vi "TempSim SubVI.vi"(0 "Stopped Boolean":refnum<vi>, 1 "Temperature Queue in":refnum<queue>, 2 "Frequency":dbl, 5 "error in (no error)":errorcluster, 6 "LightCases in":T1, 7 "Temperatures in":T4, 8 "TemperatureData in":T2) -> (10 "TemperatureData out":T2, 11 "Stop loop?":bool, 12 "LightCases out":T1, 13 "Temperatures out":T4, 14 "F0 Temp Chart":dbl(graph), 15 "F0 Gain":dbl, 16 "Kinti hõmérséklet":dbl, 17 "F1 Temp Chart":dbl(graph), 18 "F1 Gain":dbl, 19 "error out":errorcluster)   [LabVIEW 2014]
uses:
  Types/TemperatureArray.ctl
  Types/TemperatureControlData.ctl
  Types/HeatingMode.ctl
  Types/LightCases.ctl
  Types/FVGFuncts.ctl
  <vilib>/express/express arith-compare/Formula/XNode/ExpressFormulaBlockNode.xnode
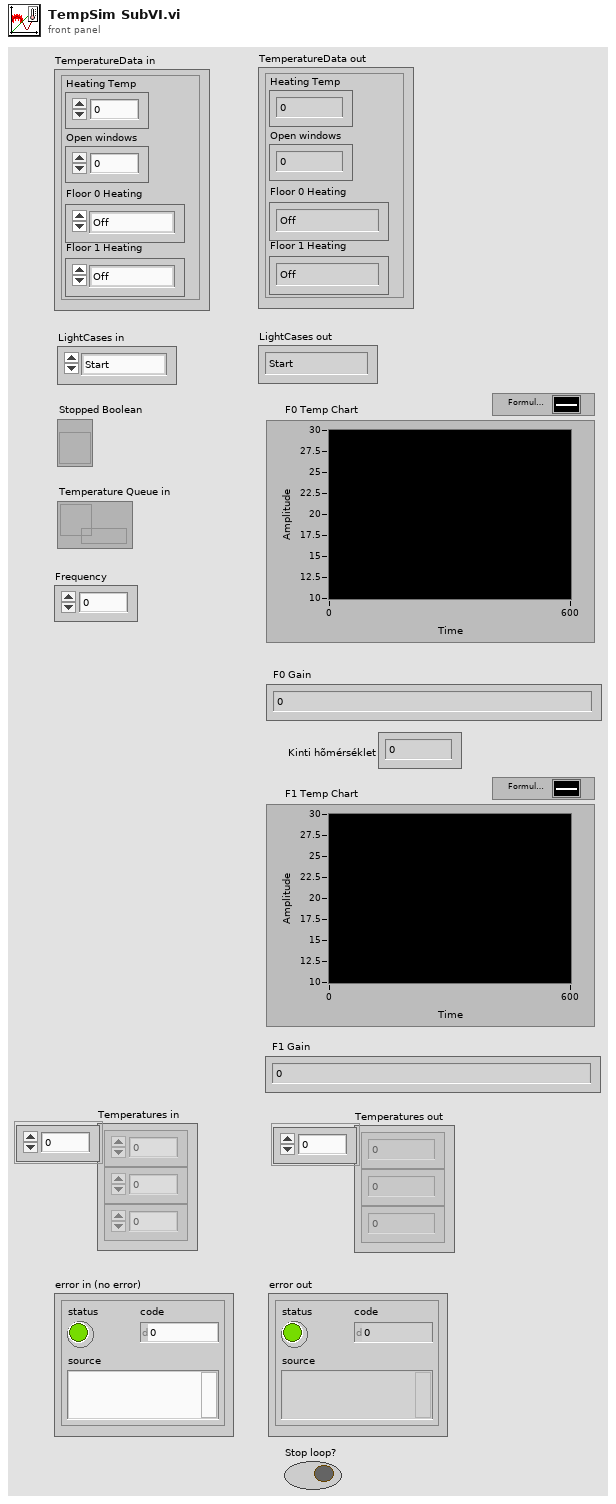
[diagram p1: front panel]
types:
  T1 = typedef "LightCases.ctl" = enum16{"Start", "Update", "Stop"}
  T2 = typedef "TemperatureControlData.ctl" = cluster{"Open windows":dbl, "Floor 0 Heating":T3, "Floor 1 Heating":T3, "Heating Temp":dbl}
  T3 = typedef "HeatingMode.ctl" = enum16{"Off", "Heating", "Cooling"}
  T4 = typedef "TemperatureArray.ctl" = dbl[]
  T5 = typedef "FVGFuncts.ctl" = enum16{"Init", "Set Data", "Get Data"}
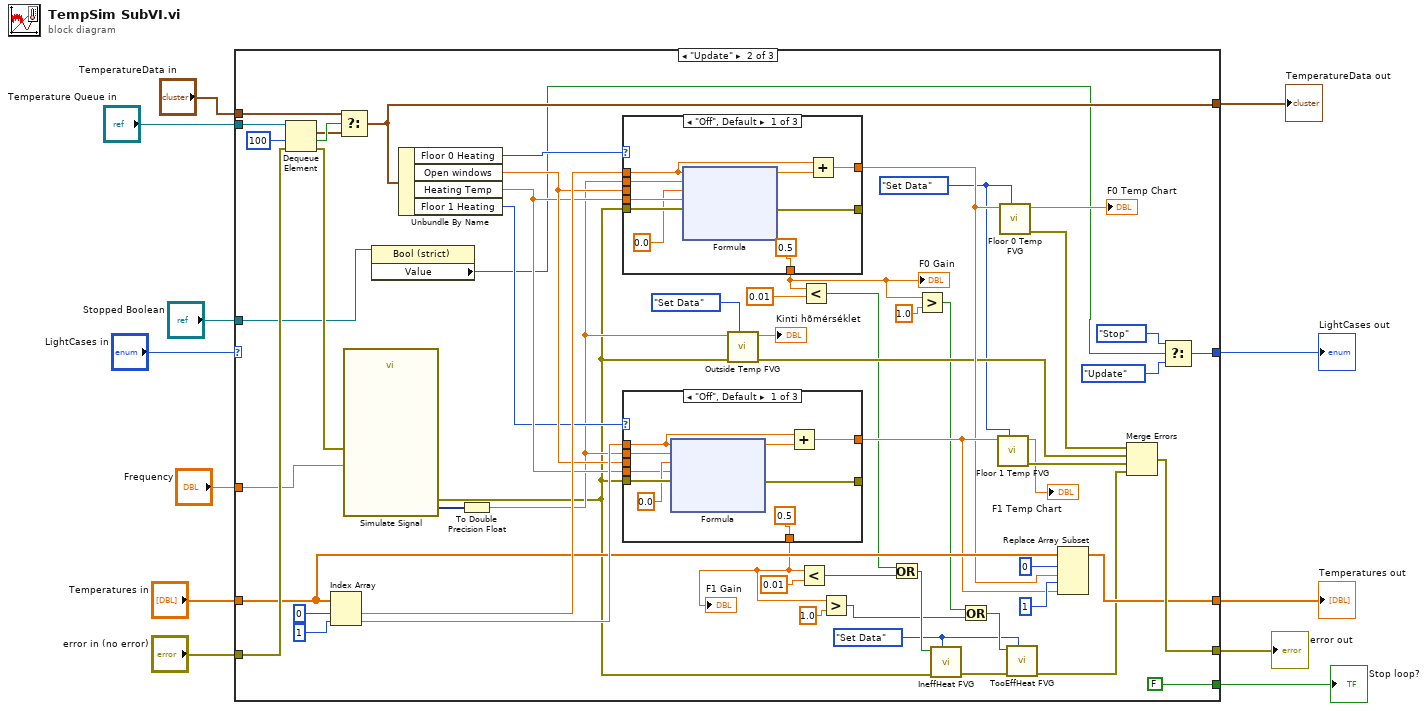
[diagram p0: block diagram]
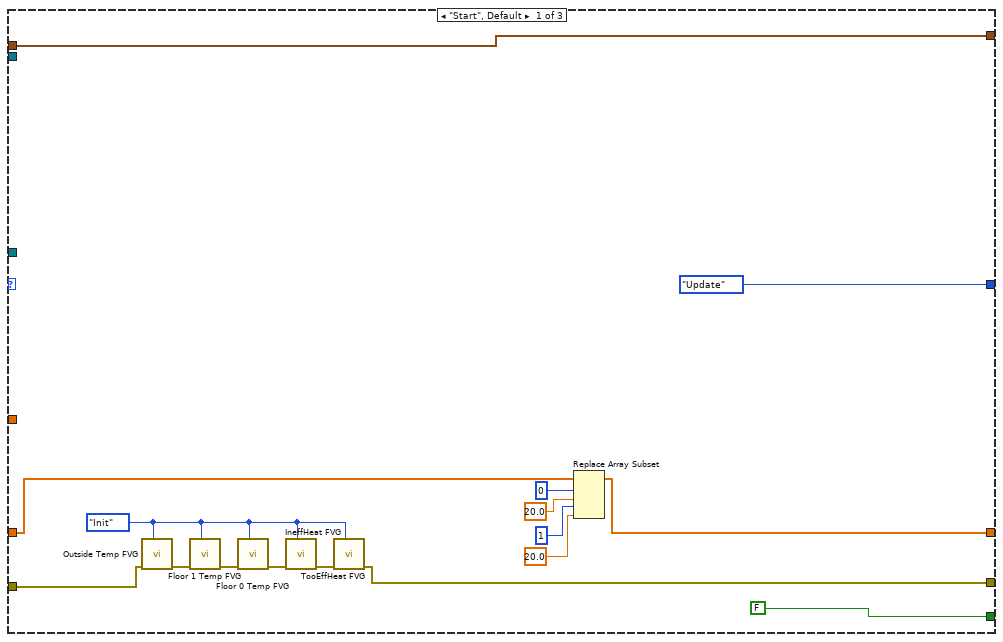
[diagram p2: hidden frame]
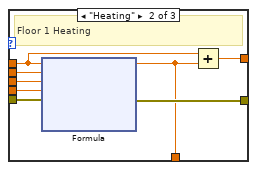
[diagram p3: hidden frame]
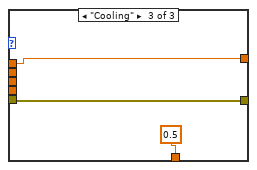
[diagram p4: hidden frame]
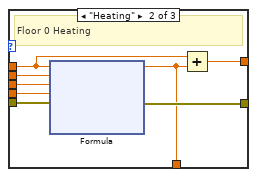
[diagram p5: hidden frame]
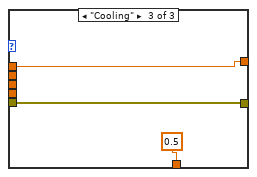
[diagram p6: hidden frame]
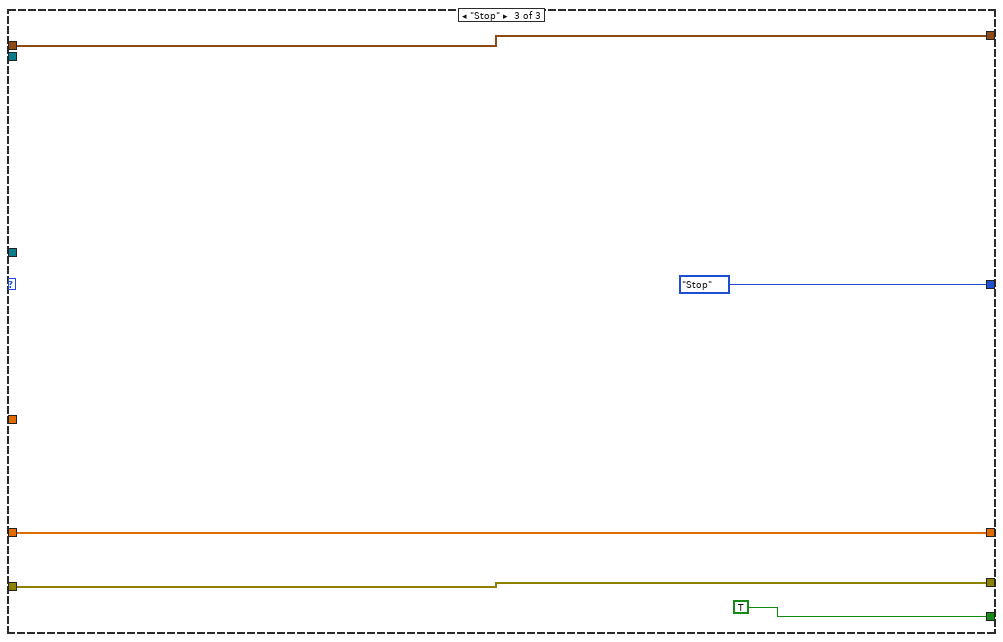
[diagram p7: hidden frame]
diagram:
  n1 = case shown="\"Update\"" "LightCases in" {
    tunnel: "Temperature Queue in" -> [_ w83 _]
    tunnel: "error in (no error)" -> [w14 w82 w182]
    tunnel: [FALSE FALSE TRUE] -> w2
    tunnel: [LightCases."Update" w74 LightCases."Stop"] -> w4
    tunnel: "TemperatureData in" -> [w26 w80 w185]
    tunnel: [w26 w62 w185] -> w6
    tunnel: [w13 w72 w182] -> w10
    tunnel: "Frequency" -> [_ w73 _]
    tunnel: "Temperatures in" -> [w25 w64 w181]
    tunnel: [w20 w63 w181] -> w8
    tunnel: "Stopped Boolean" -> [_ w30 _]
    frame "Start", Default {
      w15 = FVGFuncts."Init" ("Enum")
      n2 = call "Outside Temp FVG.vi"("Mode"=w15, "Error In"=w14) -> ("Error Out"=w18:errorcluster)  [unwired: 8 in, 1 out]
      n3 = call "Floor 1 Temp FVG.vi"("Mode"=w15, "Error In"=w18) -> ("Error Out"=w19:errorcluster)  [unwired: 8 in, 1 out]
      n4 = call "Floor 0 Temp FVG.vi"("Mode"=w15, "Error In"=w19) -> ("Error Out"=w17:errorcluster)  [unwired: 8 in, 1 out]
      n5 = call "IneffHeat FVG.vi"("Mode"=w15, "Error In"=w17) -> ("Error Out"=w16:errorcluster)  [unwired: 8 in, 1 out]
      n6 = call "TooEffHeat FVG.vi"("Mode"=w15, "Error In"=w16) -> ("Error Out"=w13:errorcluster)  [unwired: 8 in, 1 out]
      n7 = Replace Array Subset(array=w25, new element #1=20.0 ("new element/subarray"), index #1=0 ("index"), new element #2=20.0 ("new element/subarray"), index #2=1 ("index")) -> (w20:T4)
    }
    frame "Update" {
      w31 = FVGFuncts."Set Data" ("Mode")
      w36 = FVGFuncts."Set Data" ("Enum")
      n8 = Dequeue Element(queue=w83, timeout in ms (-1)=100, error in (no error)=w82) -> (element=w78:T2, timed out?=w79:bool, error out=w77:errorcluster)  [unwired: 1 out]
      n9 = Index Array(array=w64, index #1=0 ("index"), index #2=1 ("index")) -> (element #1=w67:dbl, element #2=w66:dbl)
      n10 = Select(t=w80, s=w79, f=w78) -> (s? t:f=w62:T2)
      n11 = call "Simulate Signal"("Frequency"=w73, "error in (no error)"=w77) -> ("Outside temperature"=w65:dynamicdata, "error out"=w43:errorcluster)  [unwired: 12 in]
      n12 = property class="Bool (strict)"(reference=w30) -> ("Value"=w29:bool)  [unwired: 1 in, 2 out]
      n13 = Unbundle By Name(w62) -> ("Floor 0 Heating"=w61:T3, "Open windows"=w60:dbl, "Heating Temp"=w59:dbl, "Floor 1 Heating"=w58:T3)
      n14 = To Double Precision Float(number=w65) -> (double precision float=w51:dbl)
      n15 = case shown="\"Off\", Default" w61 {
        tunnel: [w137 w163 w180] -> _
        tunnel: w43 -> [w141 w162 w180]
        tunnel: w67 -> [w133 w157 w179]
        tunnel: w51 -> [w138 w161 _]
        tunnel: w60 -> [_ w160 _]
        tunnel: w59 -> [w140 w159 _]
        tunnel: [w135 w158 w179] -> w55
        tunnel: [0.5 ("Result") w156 0.5 ("Result")] -> w38
        frame "Off", Default {
          n16 = xnode "Formula"("T_szoba"=w133, "T_kint"=w138, "H_on"=0.0, "T_h"=w140, "error in (no error)"=w141) -> ("Result"=w134:dbl, "error out"=w137:errorcluster)
          n17 = Add(x=w133, y=w134) -> (x+y=w135:dbl)
        }
        frame "Heating" {
          # "Floor 0 Heating"
          n18 = xnode "Formula"("T_szoba"=w157, "T_kint"=w161, "H_on"=w160, "T_h"=w159, "error in (no error)"=w162) -> ("Result"=w156:dbl, "error out"=w163:errorcluster)
          n19 = Add(x=w157, y=w156) -> (x+y=w158:dbl)
        }
        frame "Cooling" {
        }
      }
      "F0 Gain" <- w38
      n20 = case shown="\"Off\", Default" w58 {
        tunnel: [w89 w115 w131] -> _
        tunnel: w43 -> [w93 w114 w131]
        tunnel: w66 -> [w87 w110 w132]
        tunnel: w51 -> [w90 w113 _]
        tunnel: [w85 w109 w132] -> w57
        tunnel: w60 -> [_ w112 _]
        tunnel: w59 -> [w91 w111 _]
        tunnel: [0.5 ("Result") w108 0.5 ("Result")] -> w33
        frame "Off", Default {
          n21 = xnode "Formula"("T_szoba"=w87, "T_kint"=w90, "H_on"=0.0, "T_h"=w91, "error in (no error)"=w93) -> ("Result"=w86:dbl, "error out"=w89:errorcluster)
          n22 = Add(x=w87, y=w86) -> (x+y=w85:dbl)
        }
        frame "Heating" {
          # "Floor 1 Heating"
          n23 = xnode "Formula"("T_szoba"=w110, "T_kint"=w113, "H_on"=w112, "T_h"=w111, "error in (no error)"=w114) -> ("Result"=w108:dbl, "error out"=w115:errorcluster)
          n24 = Add(x=w110, y=w108) -> (x+y=w109:dbl)
        }
        frame "Cooling" {
        }
      }
      "F1 Gain" <- w33
      n25 = call "Outside Temp FVG.vi"("Mode"=FVGFuncts."Set Data" ("Enum"), "Error In"=w43, "Data In"=w51) -> ("Error Out"=w52:errorcluster, "Data Out"=→"Kinti hõmérséklet":dbl)  [unwired: 7 in]
      n26 = Less?(x=w33, y=0.01) -> (x < y?=w46:bool)
      n27 = Less?(x=w38, y=0.01) -> (x < y?=w45:bool)
      n28 = Greater?(x=w33, y=1.0) -> (0:w32:bool)
      n29 = Or(x=w45, y=w46) -> (x .or. y?=w42:bool)
      n30 = Greater?(x=w38, y=1.0) -> (0:w35:bool)
      n31 = call "IneffHeat FVG.vi"("Mode"=w31, "Error In"=w43, "Data In"=w42) -> ("Error Out"=w40:errorcluster)  [unwired: 7 in, 1 out]
      n32 = Or(x=w35, y=w32) -> (x .or. y?=w39:bool)
      n33 = call "Floor 1 Temp FVG.vi"("Mode"=w36, "Data In"=w57) -> ("Error Out"=w56:errorcluster, "Data Out"=→"F1 Temp Chart":dbl)  [unwired: 8 in]
      n34 = call "Floor 0 Temp FVG.vi"("Mode"=w36, "Data In"=w55) -> ("Error Out"=w53:errorcluster, "Data Out"=→"F0 Temp Chart":dbl)  [unwired: 8 in]
      n35 = call "TooEffHeat FVG.vi"("Mode"=w31, "Error In"=w40, "Data In"=w39) -> ("Error Out"=w41:errorcluster)  [unwired: 7 in, 1 out]
      n36 = Replace Array Subset(array=w64, new element #1=w55, index #1=0 ("index"), new element #2=w57, index #2=1 ("index")) -> (w63:T4)
      n37 = Merge Errors(w53, w52, w56, w41) -> (w72:errorcluster)
      n38 = Select(t=LightCases."Stop", s=w29, f=LightCases."Update") -> (s? t:f=w74:T1)
    }
    frame "Stop" {
    }
  }
  "error out" <- w10
  "Temperatures out" <- w8
  "TemperatureData out" <- w6
  "LightCases out" <- w4
  "Stop loop?" <- w2
